vi "3458A Read Stream.vi"(7 "read timeout [ms] (30000s)":u32=30000, 8 "error in (no error)":errorcluster, 9 "sample size [B]":i32=2, 10 "samples count":i32, 11 "VISA session":refnum<visa-resource-name>) -> (0 "error out":errorcluster, 1 "waveform data int32":i32[](array[numeric]), 2 "waveform data [V]":dbl[](array[numeric]), 3 "dup VISA session":refnum<visa-resource-name>, 4 "scale factor":dbl, 6 "read samples":i32)   [LabVIEW 2020, in "3458A Virtual Digitizer.lvlib" / "3458A Digitizing Low Levels.lvlib"]
doc: "Reads digitized data from memory. If 'Max Read' is set to -1 it reads all available data. It should work with SINt, DINT, SREAL and DREAL modes. ASCII read mode is not finished. It selects the OFORMAT automaticlaly. Data are returned already scaled if transfered in INT."
uses:
  3458A Digitizing Low Levels.lvlib
  3458A Basic Driver/3458A Basic Driver.lvlib
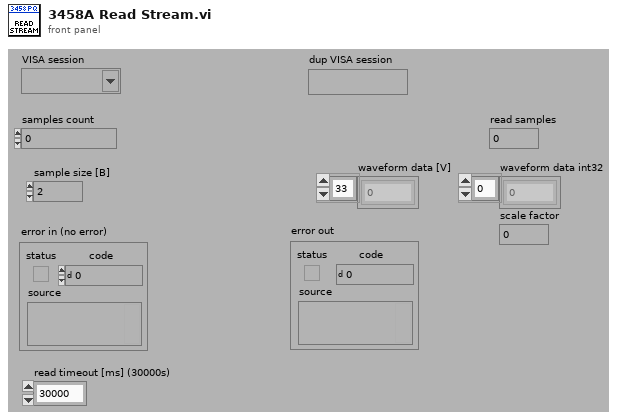
[diagram p1: front panel]
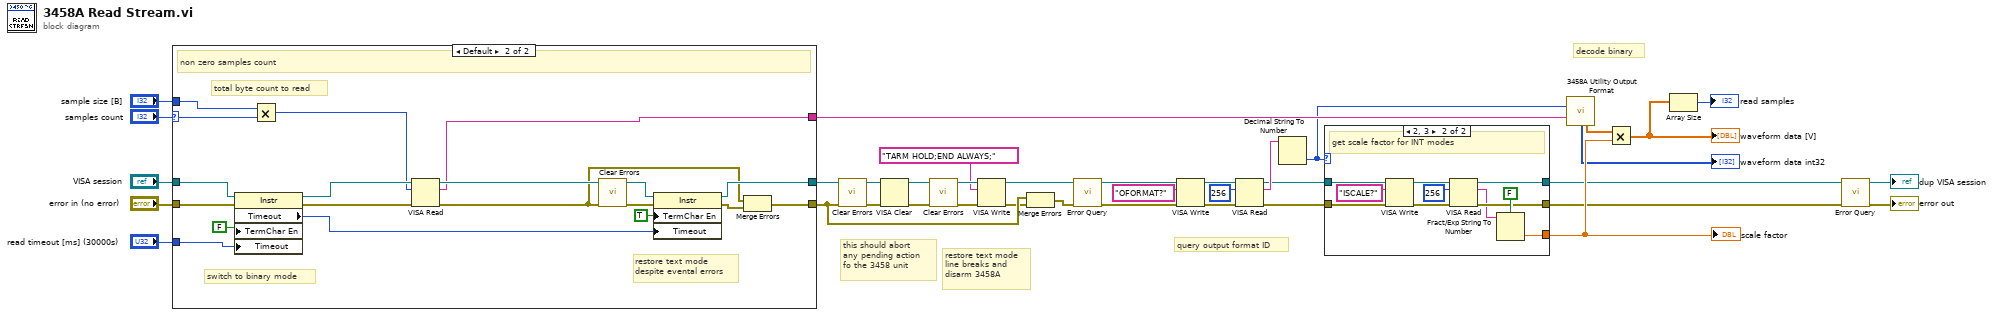
[diagram p0: block diagram]
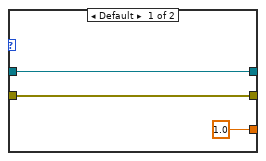
[diagram p2: hidden frame]
diagram:
  # "decode binary"
  # "query output format ID"
  # "restore text mode\nline breaks and\ndisarm 3458A"
  # "this should abort\nany pending action\nfo the 3458 unit"
  n1 = case shown="Default" "samples count" {
    selector: "samples count" -> [_ w49]
    tunnel: "VISA session" -> [w36 w55]
    tunnel: "error in (no error)" -> [w37 w54]
    tunnel: "sample size [B]" -> [_ w53]
    tunnel: "read timeout [ms] (30000s)" -> [_ w52]
    tunnel: [w37 w51] -> w17
    tunnel: [w36 w50] -> w32
    tunnel: [_ w38] -> w31
    frame 0 {
    }
    frame Default {
      # "restore text mode\ndespite evental errors"
      # "switch to binary mode"
      # "total byte count to read"
      # "non zero samples count"
      n2 = property on="Property Node" class="Instr"(reference=w55, error in=w54, "TermChar En"=FALSE, "Timeout"=w52) -> (reference out=w47:refnum<visa-resource-name>, error out=w46:errorcluster, "Timeout"=w43:u32)
      n3 = Multiply(x=w53, y=w49) -> (x*y=w39:i32)
      n4 = VISA Read(VISA resource name=w47, byte count=w39, error in (no error)=w46) -> (VISA resource name out=w44:refnum<visa-resource-name>, read buffer=w38:string, error out=w40:errorcluster)  [unwired: 1 out]
      n5 = call <vilib>:"Clear Errors.vi"("error in (no error)"=w40) -> ("error out"=w42:errorcluster)  [unwired: 5 in, 1 out]
      n6 = property class="Instr"(reference=w44, error in=w42, "TermChar En"=TRUE, "Timeout"=w43) -> (reference out=w50:refnum<visa-resource-name>, error out=w41:errorcluster)
      n7 = Merge Errors(w40, w41) -> (w51:errorcluster)
    }
  }
  n8 = call <vilib>:"Clear Errors.vi"("error in (no error)"=w17) -> ("error out"=w22:errorcluster)  [unwired: 5 in, 1 out]
  n9 = VISA Clear(VISA resource name=w32, error in (no error)=w22) -> (VISA resource name out=w19:refnum<visa-resource-name>, error out=w21:errorcluster)
  n10 = call <vilib>:"Clear Errors.vi"("error in (no error)"=w21) -> ("error out"=w20:errorcluster)  [unwired: 5 in, 1 out]
  n11 = VISA Write(VISA resource name=w19, write buffer="TARM HOLD;END ALWAYS;", error in (no error)=w20) -> (VISA resource name out=w10:refnum<visa-resource-name>, error out=w16:errorcluster)  [unwired: 1 out]
  n12 = Merge Errors(w17, w16) -> (w11:errorcluster)
  n13 = call "Error Query.vi"("error in (no error)"=w11, "VISA resource name"=w10) -> ("error out"=w9:errorcluster, "VISA resource name out"=w8:refnum<visa-resource-name>)  [unwired: 6 in, 2 out]
  n14 = VISA Write(VISA resource name=w8, write buffer="OFORMAT?", error in (no error)=w9) -> (VISA resource name out=w14:refnum<visa-resource-name>, error out=w15:errorcluster)  [unwired: 1 out]
  n15 = VISA Read(VISA resource name=w14, byte count=u32 256, error in (no error)=w15) -> (VISA resource name out=w5:refnum<visa-resource-name>, read buffer=w7:string, error out=w6:errorcluster)  [unwired: 1 out]
  n16 = Decimal String To Number(string=w7) -> (number=w4:i32)  [unwired: 2 in, 1 out]
  n17 = case shown="2, 3" w4 {
    tunnel: [w57 w64] -> w24
    tunnel: [w58 w63] -> w23
    tunnel: w5 -> [w58 w62]
    tunnel: w6 -> [w57 w61]
    tunnel: [1.0 w59] -> w28
    frame Default {
    }
    frame 2, 3 {
      # "get scale factor for INT modes"
      n18 = VISA Write(VISA resource name=w62, write buffer="ISCALE?", error in (no error)=w61) -> (VISA resource name out=w67:refnum<visa-resource-name>, error out=w66:errorcluster)  [unwired: 1 out]
      n19 = VISA Read(VISA resource name=w67, byte count=u32 256, error in (no error)=w66) -> (VISA resource name out=w63:refnum<visa-resource-name>, read buffer=w60:string, error out=w64:errorcluster)  [unwired: 1 out]
      n20 = Fract/Exp String To Number(use system decimal point (T)=FALSE, string=w60) -> (number=w59:dbl)  [unwired: 2 in, 1 out]
    }
  }
  "scale factor" <- w28
  n21 = call "3458A Utility Output Format.vi"("Output Format (0:ASCII)"=w4, "Input String"=w31) -> ("binary converted to int32"=→"waveform data int32":i32[], "anything converted to double"=w30:dbl[])  [unwired: 7 in, 5 out]
  n22 = Multiply(x=w30, y=w28) -> (x*y=w2:dbl[])
  "waveform data [V]" <- w2
  n23 = Array Size(array=w2) -> (size(s)=→"read samples":i32)
  n24 = call "Error Query.vi"("error in (no error)"=w24, "VISA resource name"=w23) -> ("error out"=→"error out":errorcluster, "VISA resource name out"=→"dup VISA session":refnum<visa-resource-name>)  [unwired: 6 in, 2 out]
